vi "Run Test Bench Linux x64.vi"() -> ()   [LabVIEW 2026]
uses:
  <userlib>/Custom Device Test Bench/Types/RT Driver States.ctl
  <vilib>/Platform/TimedLoop/XDataNode/timing_clust.ctl
  <vilib>/Platform/TimedLoop/XDataNode/nitl_modes.ctl
  <vilib>/Platform/TimedLoop/XDataNode/wakeup.ctl
  <vilib>/platform/TimedLoop/XDataNode/XDataNode.xnode
  <vilib>/Platform/TimedLoop/XDataNode/XDNodeRunTimeDep.lvlib
  Program Files/NI/LVAddons/nivscustomdeviceexpress/1/Targets/NI/RT/Linux/PXI/user.lib/Custom Devie Test Bench/Custom Device Test Bench.lvlib
panel:
  in  "Status":string="Idle. Click START to run the Test Bench ..."
  in  "Custom Device JSON File Path":path
  in  "Custom Device Test Hooks PPL Path":path
  in  "Exit":bool
  in  "Stop":bool
  in  "Start":bool
  # "-> START will run the Test Bench with user provided file path control values. \nTest Bench calls Read and Write states in a loop until user clicks STOP or EXIT\nThis would also hit any breakpoints placed in Engine code for debugging.\n\n-> STOP stops already running Test Bench execution. User's can change\nthe file path control values and click START to run the test bench with new\nvalues. \n\n-> EXIT stops any running Test Bench execution and exits the VI"
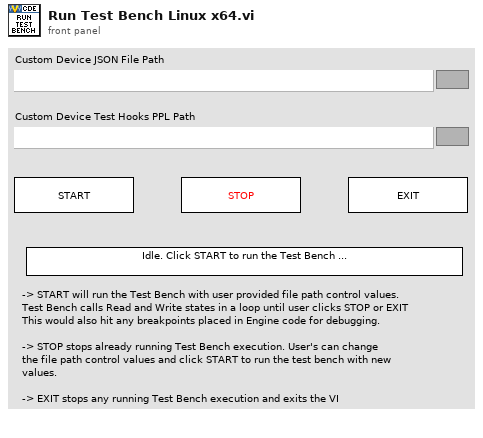
[diagram p1: front panel]
types:
  T1 = typedef "Custom Device Test Bench.lvlib/RT Driver States.ctl" = enum16{"Initialize", "Start", "Read Data from HW", "Write Data to HW", "Close"}
  T2 = typedef "XDNodeRunTimeDep.lvlib/timing_clust.ctl" = cluster{"Expected End [f-1]":u64, "Actual End [f-1]":u64, "Finished Late? [f-1]":bool, "Expected End [i-1]":u64, "Actual End [i-1]":u64, "Finished Late? [i-1]":bool, "Expected Start [i]":u64, "Actual Start [i]":u64, "Expected Start [f]":u64, "Actual Start [f]":u64, "Source Name":string, "Structure Name":string, "Period":i64, "Deadline":i64, "Offset":i64, "Start":i64, "Priority":i32, "Timeout":i32, "Mode":T3, "Wakeup Reason":T4, "Error":errorcluster, "Source Type":string, "Secondary Source Type":string, "Global End Time":u64, "Global Start Time":u64, "Frame Duration":u64, "Iteration Duration":u64, "Assigned CPU":i32, "I/O Scan Engine Mode":u32}
  T3 = typedef "XDNodeRunTimeDep.lvlib/nitl_modes.ctl" = enum32{"No Change", "Process missed periods, maintain original phase", "Discard missed periods, maintain original phase", "Process missed periods, ignore original phase", "Discard missed periods, ignore original phase"}
  T4 = typedef "XDNodeRunTimeDep.lvlib/wakeup.ctl" = enum32{"Normal", "Aborted", "Asynchronous wakeup", "Timing source error", "Timed loop error", "Timeout"}
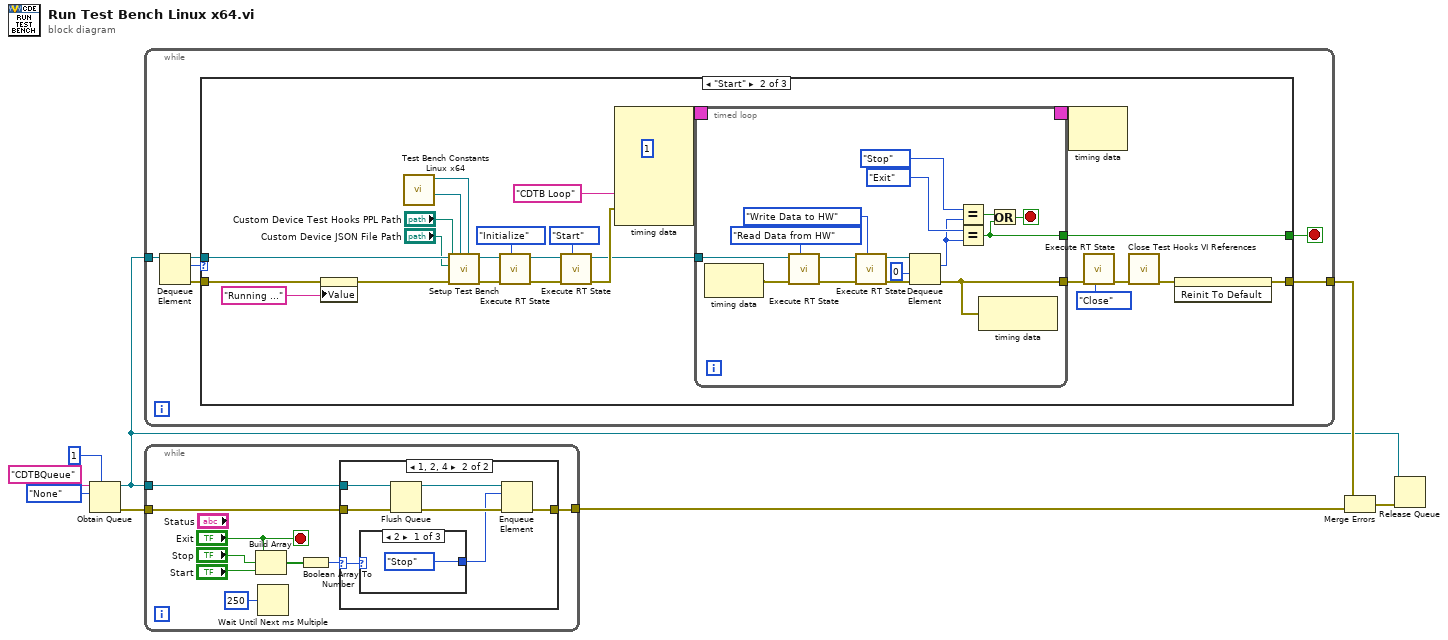
[diagram p0: block diagram]
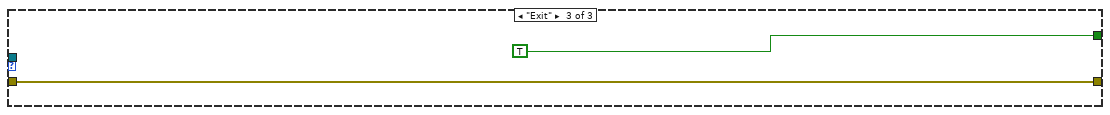
[diagram p3: hidden frame]
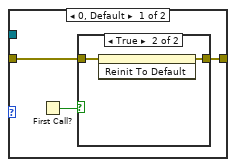
[diagram p4: hidden frame]
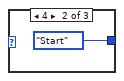
[diagram p6: hidden frame]
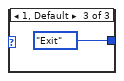
[diagram p7: hidden frame]
diagram:
  n1 = Obtain Queue(max queue size (-1, unlimited)=1, name (unnamed)="CDTBQueue", element data type=enum16{"None", "Start", "Stop", "Exit"}."None") -> (queue out=w1:refnum<queue>, error out=w8:errorcluster)  [unwired: 2 in, 1 out]
  n2 = while {
    tunnel: w1 -> [w12]
    tunnel: [w14] -> w7
    stop <- w9 stop-if-true
    n3 = Dequeue Element(queue=w12) -> (queue out=w10:refnum<queue>, element=w11:enum16{"None", "Start", "Stop", "Exit"}, error out=w13:errorcluster)  [unwired: 2 in, 1 out]
    n4 = case shown="\"Start\"" w11 {
      tunnel: w10 -> [_ w28 _]
      tunnel: [_ w27 TRUE] -> w9
      tunnel: [w15 w18 w65] -> w14
      tunnel: w13 -> [w15 w21 w65]
      frame "None", Default {
      }
      frame "Start" {
        n5 = property on="Status" class="Str"(error in=w21, "Value"="Running ...") -> (error out=w22:errorcluster)  [unwired: 1 in, 1 out]
        n6 = call "Test Bench Constants Linux x64.vi"() -> ("Deployment Hooks class"=w16:refnum<class "Custom Device Deployment Hooks.lvclass">, "Custom Device class"=w17:refnum<class "Custom Device.lvclass">)  [unwired: 10 in]
        n7 = call "Setup Test Bench.vi"("Custom Device class"=w17, "Development Hooks class"=w16, "error in"=w22, "JSON path"="Custom Device JSON File Path", "Custom Device Test Hooks PPL Path"="Custom Device Test Hooks PPL Path") -> ("error out"=w36:errorcluster)  [unwired: 6 in]
        n8 = call <userlib>:"Execute RT State.vi"("RT Driver States"=RT_Driver_States."Initialize", "error in"=w36) -> ("error out"=w38:errorcluster)  [unwired: 9 in]
        n9 = call <userlib>:"Execute RT State.vi"("RT Driver States"=RT_Driver_States."Start", "error in"=w38) -> ("error out"=w37:errorcluster)  [unwired: 9 in]
        n10 = node-c288(i64 1 ("Period"), "CDTB Loop" ("Structure Name"), w37) -> (w34:T2)  [unwired: 3 in]
        n11 = timed-loop {
          timing: w34 -> [_]
          timing-out: [_] -> w33
          tunnel: [w49] -> w20
          tunnel: w28 -> [w46]
          tunnel: [w40] -> w27
          stop <- w39 stop-if-true
          n12 = node-c288() -> (w51:errorcluster)  [unwired: 1 in]
          n13 = call <userlib>:"Execute RT State.vi"("RT Driver States"=RT_Driver_States."Read Data from HW", "error in"=w51) -> ("error out"=w52:errorcluster)  [unwired: 9 in]
          n14 = call <userlib>:"Execute RT State.vi"("RT Driver States"=RT_Driver_States."Write Data to HW", "error in"=w52) -> ("error out"=w50:errorcluster)  [unwired: 9 in]
          n15 = Dequeue Element(queue=w46, timeout in ms (-1)=0, error in (no error)=w50) -> (element=w42:enum16{"None", "Start", "Stop", "Exit"}, error out=w49:errorcluster)  [unwired: 2 out]
          n16 = Equal?(x=enum16{"None", "Start", "Stop", "Exit"}."Stop" ("y"), y=w42) -> (x = y?=w41:bool)
          n17 = Equal?(x=enum16{"None", "Start", "Stop", "Exit"}."Exit" ("y"), y=w42) -> (x = y?=w40:bool)
          n18 = node-c288(w49) -> ()  [unwired: 1 out]
          n19 = Or(x=w41, y=w40) -> (x .or. y?=w39:bool)
        }
        n20 = node-c288(w33) -> ()  [unwired: 1 out]
        n21 = call <userlib>:"Execute RT State.vi"("RT Driver States"=RT_Driver_States."Close", "error in"=w20) -> ("error out"=w35:errorcluster)  [unwired: 9 in]
        n22 = call <userlib>:"Close Test Hooks VI References.vi"("error in"=w35) -> ("error out"=w19:errorcluster)  [unwired: 10 in]
        n23 = invoke on="Status" class="Str" method="Reinit To Default"(error in=w19) -> (error out=w18:errorcluster)  [unwired: 2 in, 2 out]
      }
      frame "Exit" {
      }
    }
  }
  n24 = while {
    tunnel: w1 -> [w70]
    tunnel: w8 -> [w69]
    tunnel: [w68] -> w6
    stop <- "Exit" stop-if-true
    n25 = Build Array("Exit", "Stop", "Start") -> (w72:bool[])
    n26 = Wait Until Next ms Multiple(millisecond multiple=u32 250) -> ()  [unwired: 1 out]
    n27 = Boolean Array To Number(Boolean array=w72) -> (number=w71:u32)
    n28 = case shown="1, 2, 4" w71 {
      selector: w71 -> [_ w82]
      tunnel: w70 -> [_ w87]
      tunnel: w69 -> [w76 w86]
      tunnel: [w75 w83] -> w68
      frame 0, Default {
        n29 = First Call?() -> (First Call?: T/F=w77:bool)
        n30 = case shown="True" w77 {
          tunnel: w76 -> [w78 w80]
          tunnel: [w78 w79] -> w75
          frame False {
          }
          frame True {
            n31 = invoke on="Status" class="Str" method="Reinit To Default"(error in=w80) -> (error out=w79:errorcluster)  [unwired: 2 in, 2 out]
          }
        }
      }
      frame 1, 2, 4 {
        n32 = case shown="2" w82 {
          tunnel: [enum16{"None", "Start", "Stop", "Exit"}."Stop" enum16{"None", "Start", "Stop", "Exit"}."Start" enum16{"None", "Start", "Stop", "Exit"}."Exit"] -> w81
          frame 2 {
          }
          frame 4 {
          }
          frame 1, Default {
          }
        }
        n33 = Flush Queue(queue=w87, error in (no error)=w86) -> (queue out=w85:refnum<queue>, error out=w84:errorcluster)  [unwired: 1 out]
        n34 = Enqueue Element(queue=w85, element=w81, error in (no error)=w84) -> (error out=w83:errorcluster)  [unwired: 1 in, 2 out]
      }
    }
  }
  n35 = Merge Errors(w7, w6) -> (w5:errorcluster)
  n36 = Release Queue(queue=w1, error in (no error)=w5) -> ()  [unwired: 1 in, 3 out]
